vi "get stored or default message.vi"(11 "failure in":T1 {"code" format="%.0x"}) -> (2 "message":string, 3 "failure out":T1 {"code" format="%.0x"})   [LabVIEW 2013, in "failure.lvlib"]
uses:
  failure.lvlib
  failure.ctl
  const messagename.vi
  <vilib>/Utility/error.llb/Error Code Database.vi
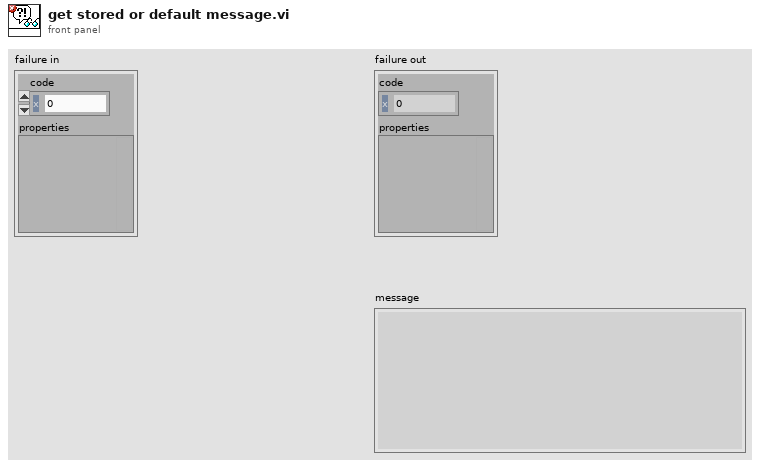
[diagram p1: front panel]
types:
  T1 = typedef "failure.lvlib/failure.ctl" = cluster{"code":i32, "properties":variant}
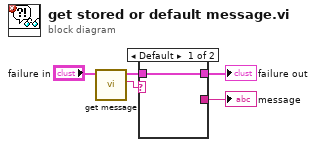
[diagram p0: block diagram]
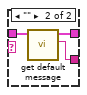
[diagram p2: hidden frame]
diagram:
  n1 = call "get message.vi"("failure in"="failure in") -> ("message"=w2:string, "failure out"=w4:T1)  [unwired: 9 in]
  n2 = case shown="Default" w2 {
    tunnel: w4 -> [w6 w9]
    tunnel: [w6 w8] -> w3
    tunnel: [_ w7] -> w1
    frame Default {
    }
    frame "" {
      n3 = call "get default message.vi"("failure in"=w9) -> ("message"=w7:string, "failure out"=w8:T1)  [unwired: 9 in]
    }
  }
  "failure out" <- w3
  "message" <- w1
